vi "Rename As Application Main.vi"() -> ()   [LabVIEW 2020]
doc: "This VI can be used as a launcher VI for the main application or as a debugging tool.\n_____\nBased on DQMH Project Template 6.1.0.94."
uses:
  Libraries/Rename As Application UI/Rename As Application UI.lvlib
  Libraries/Launcher Support/Launcher Support.lvlib
  <vilib>/Peloton/Pelobuttons/Pelobuttons_lib_Pelobuttons.lvlib
panel:
  in  "Launch UI API Tester":bool
  out "Command Line Arguments":string[](array[string])
  out "Module Running?":bool
  out "Status":string
  out "error out":errorcluster
  in  "Stop Module":bool
  in  "Start Module":bool
  # "See the Build_Final_EXE bookmarks on the diagram for instructions on using this VI as a launcher for an EXE."
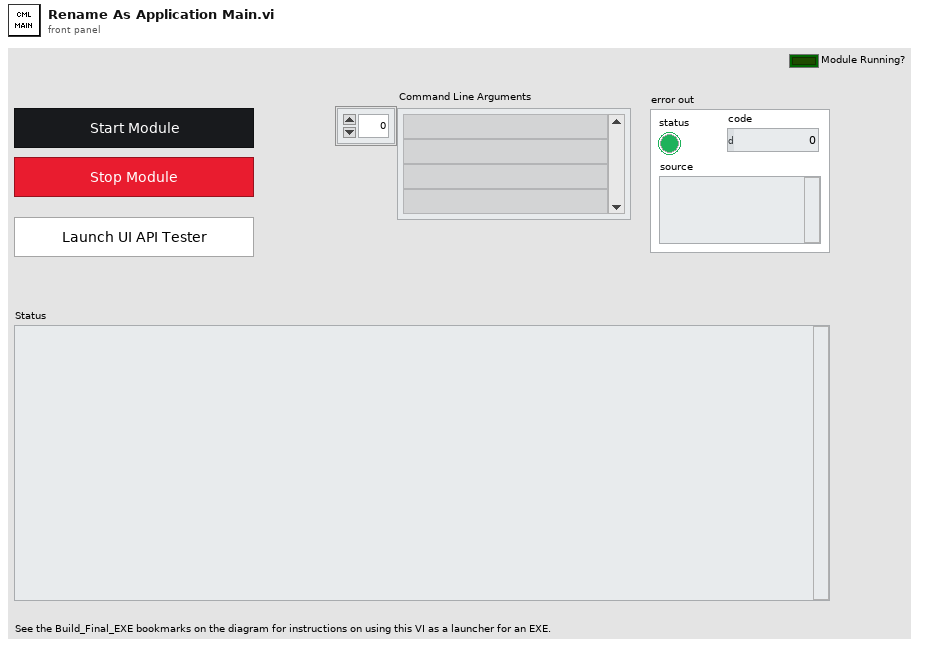
[diagram p1: front panel]
types:
  T1 = enum32{"invalid app kind", "Development System", "Run Time System", "Student Edition", "Embedded LabVIEW", "Evaluation", "Custom"}
  T2 = typedef "Rename As Application UI.lvlib/Broadcast Events--cluster.ctl" = cluster{"Module Did Init":refnum<user-event>, "Status Updated":refnum<user-event>, "Error Reported":refnum<user-event>, "Module Did Stop":refnum<user-event>, "Update Module Execution Status":refnum<user-event>}
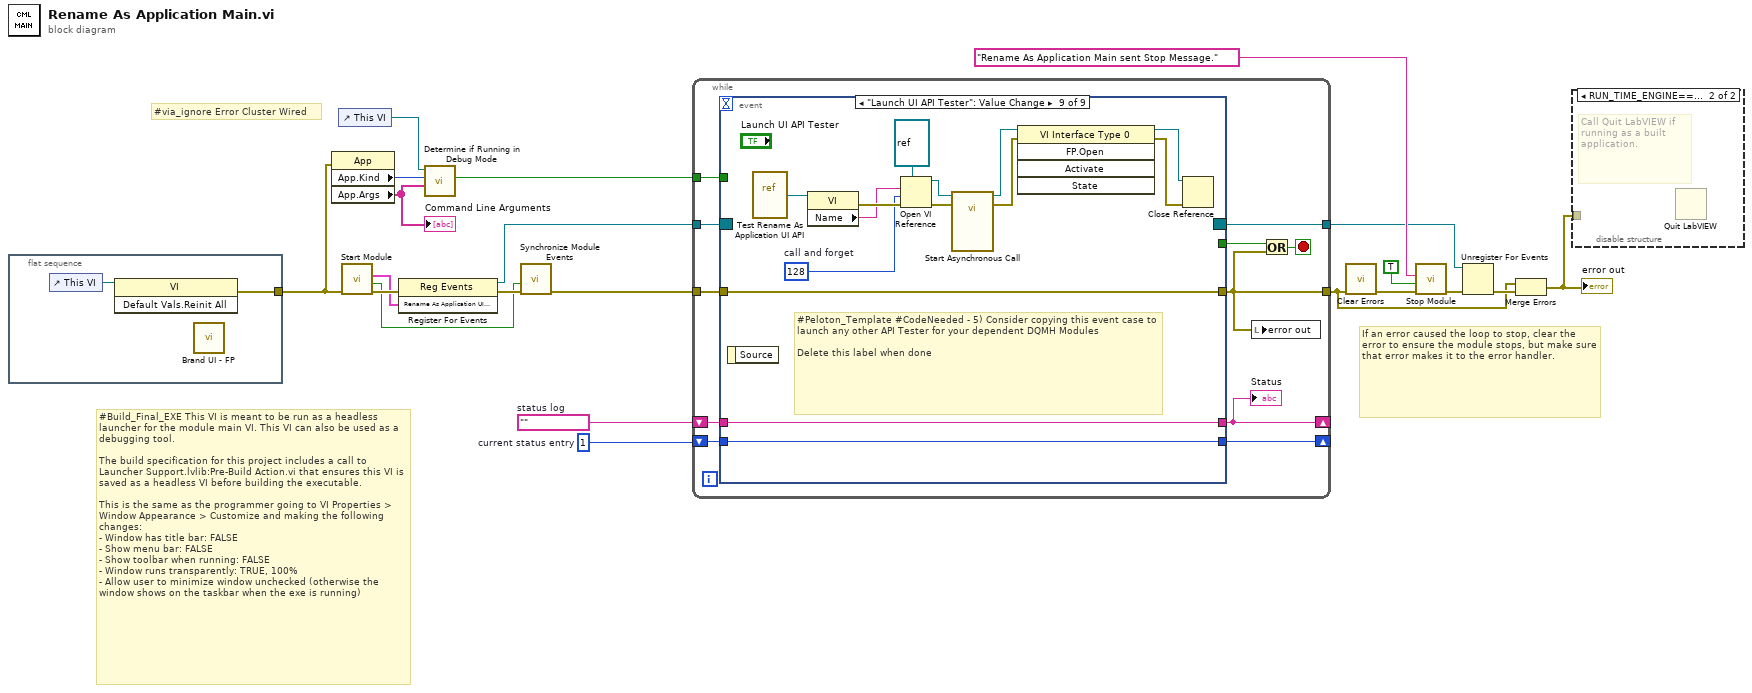
[diagram p0: block diagram]
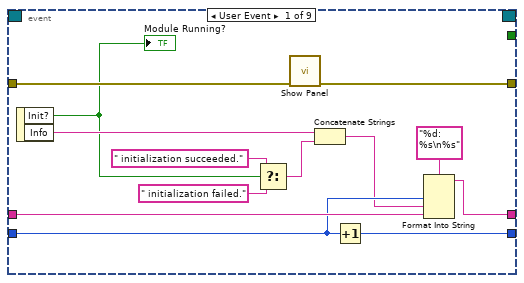
[diagram p2: hidden frame]
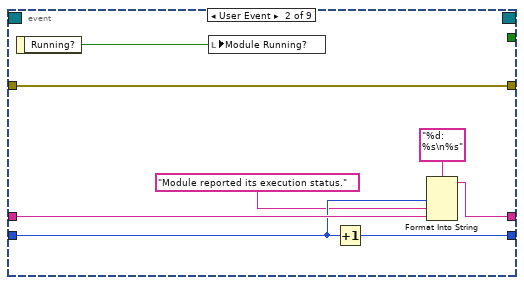
[diagram p3: hidden frame]
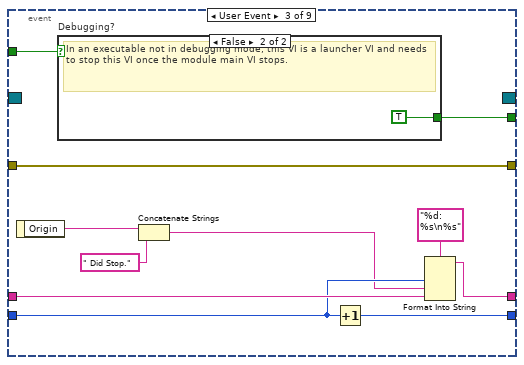
[diagram p4: hidden frame]
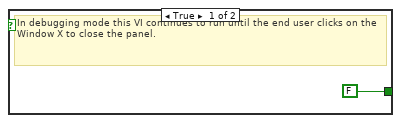
[diagram p5: hidden frame]
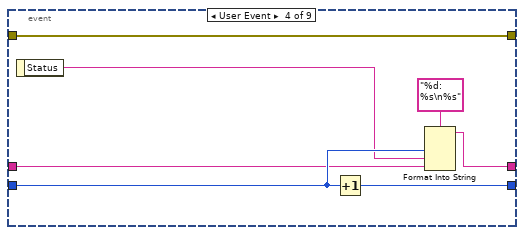
[diagram p6: hidden frame]
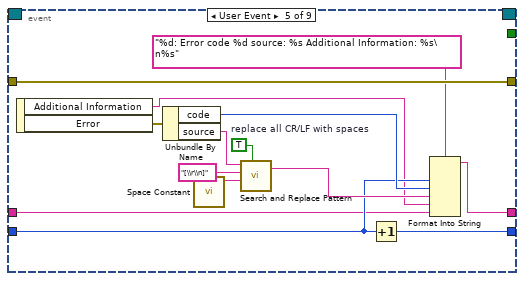
[diagram p7: hidden frame]
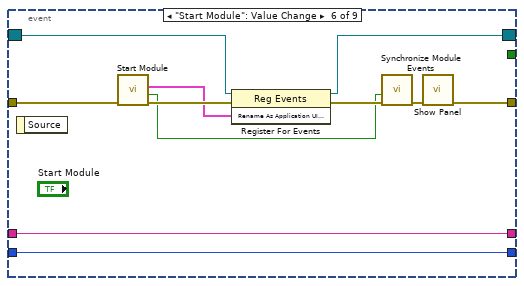
[diagram p8: hidden frame]
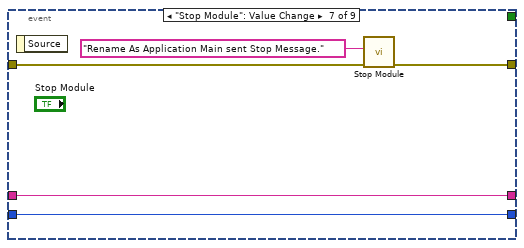
[diagram p9: hidden frame]
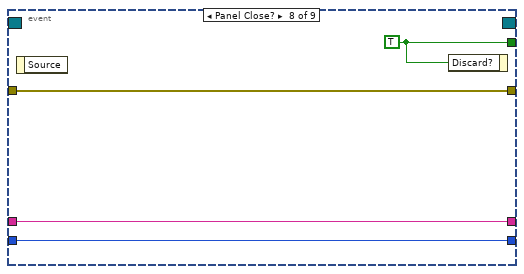
[diagram p10: hidden frame]
diagram:
  w17 = 1  # current status entry
  w18 = ""  # status log
  # "#via_ignore Error Cluster Wired"
  # "#Build_Final_EXE This VI is meant to be run as a headless launcher for the module main VI. This VI can also be used as a debugging tool. \n\nThe build specification for this project includes a call to Launcher Support.lvlib:Pre-Build Action.vi that ensures this VI is saved as a headless VI before building the executable.\n\nThis is the same as the programmer going to VI Properties > Window Appearance > Customize and making the following changes:\n- Window has title bar: FALSE\n- Show menu bar: FALSE\n- Show toolbar when running: FALSE\n- Window runs transparently: TRUE, 100%\n- Allow user to minimize window unchecked (otherwise the window shows on the taskbar when the exe is running)"
  # "If an error caused the loop to stop, clear the error to ensure the module stops, but make sure that error makes it to the error handler."
  n1 = flat-sequence {
    tunnel: [w23] -> w1
    frame #0 {
      n2 = control-ref of="This VI"() -> (w22:refnum<vi>)
      n3 = invoke on="Invoke Node" class="VI" method="Default Vals.Reinit All"(reference=w22) -> (error out=w23:errorcluster)  [unwired: 2 in, 2 out]
      n4 = call <vilib>:"Brand UI - FP.vi"() -> ()  [unwired: 12 in]
    }
  }
  n5 = property on="Property Node" class="App"(error in=w1) -> ("App.Kind"=w2:T1, "App.Args"=w5:string[])  [unwired: 1 in, 2 out]
  "Command Line Arguments" <- w5
  n6 = control-ref of="This VI"() -> (w4:refnum<vi>)
  n7 = call "Start Module.vi"("error in"=w1) -> ("error out"=w12:errorcluster, "Wait for Event Sync?"=w11:bool, "Rename As Application UI Broadcast Events"=w10:T2)  [unwired: 7 in, 1 out]
  n8 = register-events(error in=w12, w10) -> (reference out=w9:refnum<event-registration>, error out=w13:errorcluster)  [unwired: 1 in]
  n9 = call "Determine if Running in Debug Mode.vi"("App.Args"=w5, "App.Kind"=w2, "Launcher VI ref"=w4) -> ("Debug mode?"=w3:bool)  [unwired: 8 in]
  n10 = call "Synchronize Module Events.vi"("error in"=w13, "Wait for Event Sync?"=w11) -> ("error out"=w7:errorcluster)  [unwired: 9 in]
  n11 = while {
    tunnel: w9 -> [w34]
    tunnel: [w25] -> w6
    shift-right: [w26] -> _
    shift-left: w18 -> [w31]
    shift-right: [w30] -> _
    shift-left: w17 -> [w32]
    tunnel: w7 -> [w28]
    tunnel: [w27] -> w16
    tunnel: w3 -> [w24]
    stop <- w29 stop-if-true
    n12 = event shown="[8] \"Launch UI API Tester\": Value Change" {
      selector: w34 -> [_ _ _ _ _ w94 _ _ _]
      dyn-events: [_ _ _ _ _ w93 _ _ _] -> w27
      timeout: _ -> [_ _ _ _ _ _ _ _ _]
      tunnel: [_ _ w57 _ _ _ _ w109 _] -> w33
      tunnel: [w35 w49 w58 w69 w89 w90 w103 w106 w123] -> w25
      tunnel: w32 -> [w44 w53 w64 w72 w79 w97 w104 w107 w121]
      tunnel: w31 -> [w45 w54 w65 w71 w77 w98 w105 w108 w122]
      tunnel: [w42 w51 w62 w73 w80 w98 w105 w108 w122] -> w26
      tunnel: [w43 w52 w63 w75 w78 w97 w104 w107 w121] -> w30
      tunnel: w28 -> [w47 w49 w58 w69 w89 w92 w101 w106 w123]
      tunnel: w24 -> [_ _ w56 _ _ _ _ _ _]
      event User Event {
        n13 = event-data() -> ("Init?"=w39:bool, "Info"=w41:string)  [unwired: 1 in]
        "Module Running?" <- w39
        n14 = Select(t=" initialization succeeded.", s=w39, f=" initialization failed.") -> (s? t:f=w36:string)
        n15 = call "Show Panel.vi"("error in (no error)"=w47) -> ("error out"=w35:errorcluster)  [unwired: 10 in]
        n16 = Concatenate Strings(w41, w36) -> (w40:string)
        n17 = Increment(x=w44) -> (x+1=w43:i32)
        n18 = Format Into String(format string="%d: %s\n%s", w44, w40, w45) -> (resulting string=w42:string)  [unwired: 2 in, 1 out]
      }
      event User Event {
        n19 = event-data() -> ("Running?"=w48:bool)  [unwired: 1 in]
        n20 = local write "Module Running?"(w48) -> ()
        n21 = Increment(x=w53) -> (x+1=w52:i32)
        n22 = Format Into String(format string="%d: %s\n%s", w53, "Module reported its execution status.", w54) -> (resulting string=w51:string)  [unwired: 2 in, 1 out]
      }
      event User Event {
        n23 = event-data() -> ("Origin"=w61:string)  [unwired: 1 in]
        n24 = case "Debugging?" shown="False" w56 {
          tunnel: [FALSE ("Discard?") TRUE ("Discard?")] -> w57
          frame True {
            # "In debugging mode this VI continues to run until the end user clicks on the Window X to close the panel."
          }
          frame False {
            # "In an executable not in debugging mode, this VI is a launcher VI and needs to stop this VI once the module main VI stops."
          }
        }
        n25 = Concatenate Strings(w61, " Did Stop.") -> (w60:string)
        n26 = Increment(x=w64) -> (x+1=w63:i32)
        n27 = Format Into String(format string="%d: %s\n%s", w64, w60, w65) -> (resulting string=w62:string)  [unwired: 2 in, 1 out]
      }
      event User Event {
        n28 = event-data() -> ("Status"=w70:string)  [unwired: 1 in]
        n29 = Increment(x=w72) -> (x+1=w75:i32)
        n30 = Format Into String(format string="%d: %s\n%s", w72, w70, w71) -> (resulting string=w73:string)  [unwired: 2 in, 1 out]
      }
      event User Event {
        w85 = TRUE  # replace all CR/LF with spaces
        n31 = event-data() -> ("Additional Information"=w76:string, "Error"=w81:errorcluster)  [unwired: 1 in]
        n32 = Unbundle By Name(w81) -> ("code"=w82:i32, "source"=w83:string)
        n33 = call <vilib>:"Space Constant.vi"() -> ("String"=w86:string)
        n34 = call <vilib>:"Search and Replace Pattern.vi"("string"=w83, "regular expression (\"\")"="[\\r\\n]" ("regular expression (\"\")"), "replace string (\"\")"=w86, "replace all? (F)"=w85) -> ("result string"=w84:string)  [unwired: 1 in, 1 out]
        n35 = Increment(x=w79) -> (x+1=w78:i32)
        n36 = Format Into String(format string="%d: Error code %d source: %s Additional Information: %s\n%s", w79, w82, w84, w76, w77) -> (resulting string=w80:string)  [unwired: 2 in, 1 out]
      }
      event "Start Module": Value Change {
        n37 = event-data() -> ()  [unwired: 1 in, 1 out]
        n38 = call "Start Module.vi"("error in"=w92) -> ("error out"=w99:errorcluster, "Wait for Event Sync?"=w96:bool, "Rename As Application UI Broadcast Events"=w95:T2)  [unwired: 7 in, 1 out]
        n39 = register-events(reference=w94, error in=w99, w95) -> (reference out=w93:refnum<event-registration>, error out=w100:errorcluster)
        n40 = call "Synchronize Module Events.vi"("error in"=w100, "Wait for Event Sync?"=w96) -> ("error out"=w91:errorcluster)  [unwired: 9 in]
        n41 = call "Show Panel.vi"("error in (no error)"=w91) -> ("error out"=w90:errorcluster)  [unwired: 10 in]
      }
      event "Stop Module": Value Change {
        n42 = event-data() -> ()  [unwired: 1 in, 1 out]
        n43 = call "Stop Module.vi"("error in"=w101, "Origin"="Rename As Application Main sent Stop Message.") -> ("error out"=w103:errorcluster)  [unwired: 9 in]
      }
      event Panel Close? {
        w109 = TRUE ("Discard?")
        n44 = event-data() -> ()  [unwired: 1 in, 1 out]
        n45 = event-data ("Event Filter Node")("Discard?"=w109) -> ()  [unwired: 1 in, 1 out]
      }
      event "Launch UI API Tester": Value Change {
        w114 = 128  # call and forget
        # "#Peloton_Template #CodeNeeded - 5) Consider copying this event case to launch any other API Tester for your dependent DQMH Modules\n\nDelete this label when done"
        n46 = event-data() -> ()  [unwired: 1 in, 1 out]
        n47 = vi-ref "Test Rename As Application UI API.vi"() -> (w118:refnum<vi>)
        n48 = property class="VI"(reference=w118) -> (error out=w120:errorcluster, "Name"=w119:string)  [unwired: 1 in, 1 out]
        n49 = Open VI Reference(type specifier VI Refnum (for type only)=refnum<vi> refnum, vi path=w119, options=w114, error in (no error)=w120) -> (vi reference=w116:refnum<vi>, error out=w117:errorcluster)  [unwired: 2 in]
        n50 = call-by-ref "Start Asynchronous Call"(reference=w116, error in=w117) -> (reference out=w113:refnum<vi>, error out=w111:errorcluster)  [unwired: 12 in]
        n51 = invoke class="VI Interface Type 0" method="FP.Open"(reference=w113, error in=w111) -> (reference out=w112:refnum<vi>, error out=w110:errorcluster)  [unwired: 3 in, 3 out]
        n52 = Close Reference(reference=w112, error in (no error)=w110) -> ()  [unwired: 1 out]
      }
    }
    "Status" <- w26
    n53 = local write "error out"(w25) -> ()
    n54 = Or(x=w33, y=w25) -> (x .or. y?=w29:bool)
  }
  n55 = call <vilib>:"Clear Errors.vi"("error in (no error)"=w6) -> ("error out"=w14:errorcluster)  [unwired: 5 in, 1 out]
  n56 = call "Stop Module.vi"("error in"=w14, "Wait for Module to Stop? (F)"=TRUE ("Wait for Module to stop?"), "Origin"="Rename As Application Main sent Stop Message.") -> ("error out"=w20:errorcluster)  [unwired: 8 in]
  n57 = Unregister For Events(event registration refnum=w16, error in=w20) -> (error out=w21:errorcluster)
  n58 = Merge Errors(w6, w21) -> (w8:errorcluster)
  "error out" <- w8
  n59 = disable-structure "Conditional Disable Structure" shown="RUN_TIME_ENGINE==True" {
    disable-tunnel: w8 -> [_ _]
    frame condition #0 (active) {
    }
    frame condition #1 {
      # "Call Quit LabVIEW if running as a built application."
      n60 = Quit LabVIEW() -> ()  [unwired: 1 in]
    }
  }
